vi "读取二维图片.vi"(8 "error in (no error)":errorcluster caption="错误输入（无错误）", 11 "Nagivation 2.0输入":refnum<class "Nagivation 2.0.lvclass">) -> (0 "error out":errorcluster caption="错误输出", 2 "二维图片":picture, 3 "Nagivation 2.0输出":refnum<class "Nagivation 2.0.lvclass">)   [LabVIEW 2018, in "Nagivation 2.0.lvclass"]
uses:
  Nagivation 2.0.lvclass
  Nagivation 2.0.lvclass/Nagivation 2.0.ctl
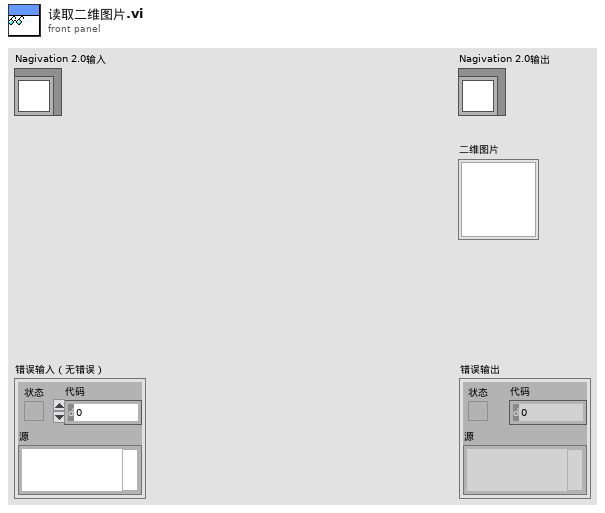
[diagram p1: front panel]
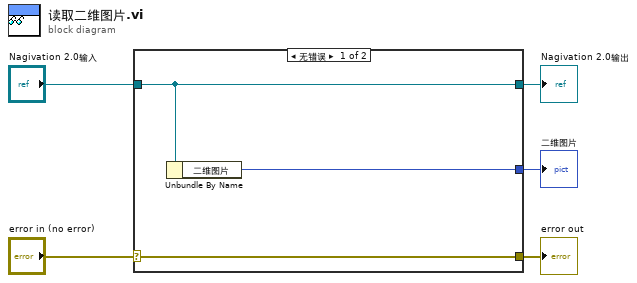
[diagram p0: block diagram]
diagram:
  n1 = case shown="无错误" "error in (no error)" {
    selector: "error in (no error)" -> [w8 w9]
    tunnel: [w8 w9] -> w4
    tunnel: [w7 w10] -> w2
    tunnel: "Nagivation 2.0输入" -> [w7 w10]
    tunnel: [w6 _] -> w1
    frame No Error {
      n2 = Unbundle By Name(w7) -> ("二维图片"=w6:picture)
    }
    frame Error {
    }
  }
  "error out" <- w4
  "Nagivation 2.0输出" <- w2
  "二维图片" <- w1
